vi "matlab_for_acquisition.vi"(4 "illumination last degree":dbl, 6 "illumination delay degree":dbl, 8 "dmd pattern num":dbl, 9 "camera delay degree":dbl, 10 "dmd delay degree":dbl, 11 "signal_time(ms)":dbl) -> (0 "exposure time":dbl, 1 "sample num":dbl, 2 "DO signal":dbl[][](array[numeric]), 3 "sample rate":dbl, 5 "dmd_picture_time":dbl)   [LabVIEW 2019]
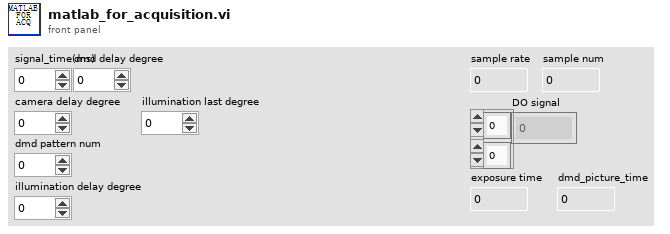
[diagram p1: front panel]
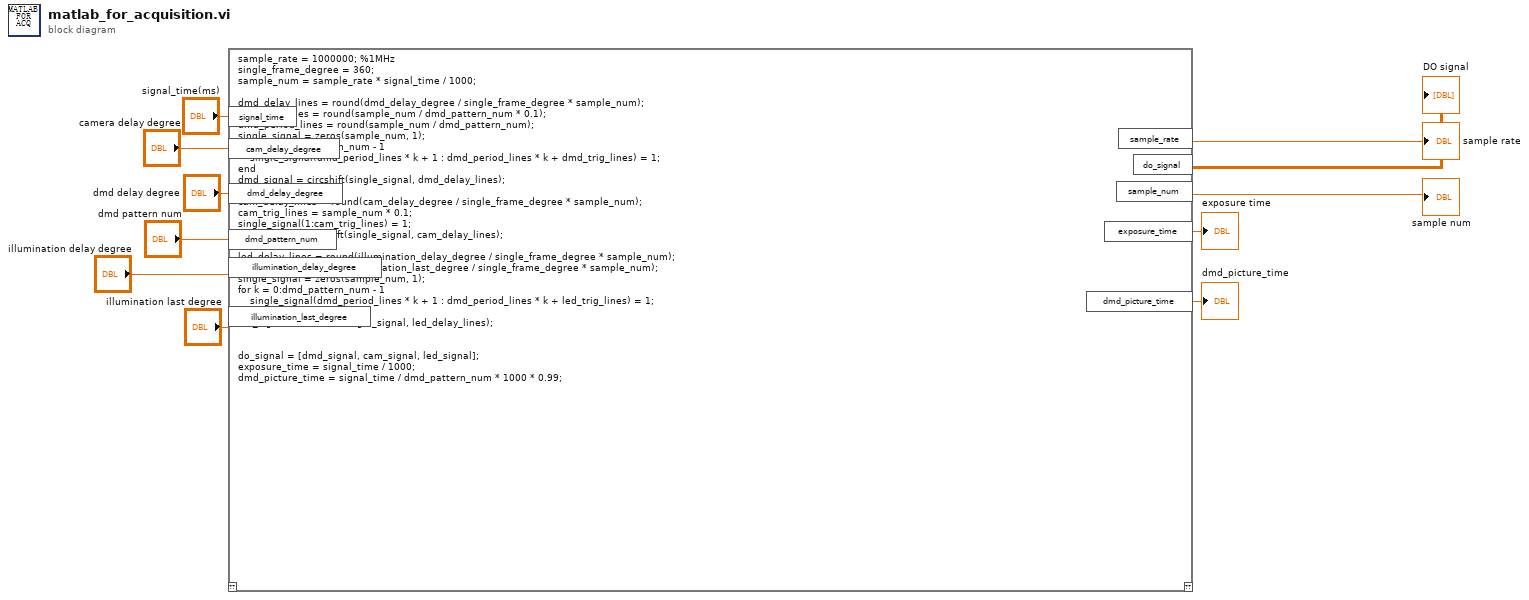
[diagram p0: block diagram]
diagram:
  n1 = script code="sample_rate = 1000000; %1MHz\nsingle_frame_degree = 360;\nsample_num = sample_rate * signal_time / 1000;\n\ndmd_delay_lines = round(dmd_delay_degree / single_frame_degree * sample_num);\ndmd_trig_lines = round(sample_num / dmd_pattern_num * 0.1);\ndmd_period_lines = round(sample_num / dmd_pattern_num);\nsingle_signal = zeros(sample_num, 1);\nfor k = 0:dmd_pattern_num - 1\n    single_signal(dmd_period_lines * k + 1 : dmd_period_lines * k + dmd_trig_lines) = 1;\nend\ndmd_signal = circshift(single_signal, dmd_delay_lines);\n\ncam_delay_lines = round(cam_delay_degree / single_frame_degree * sample_num);\ncam_trig_lines = sample_num * 0.1;\nsingle_signal(1:cam_trig_lines) = 1;\ncam_signal = circshift(single_signal, cam_delay_lines);\n\nled_delay_lines = round(illumination_delay_degree / single_frame_degree * sample_num);\nled_trig_lines = round(illumination_last_degree / single_frame_degree * sample_num);\nsingle_signal = zeros(sample_num, 1);\nfor k = 0:dmd_pattern_num - 1\n    single_signal(dmd_period_lines * k + 1 : dmd_period_lines * k + led_trig_lines) = 1;\nend\nled_signal = circshift(single_signal, led_delay_lines);\n\n\ndo_signal = [dmd_signal, cam_signal, led_signal];\nexposure_time = signal_time / 1000;\ndmd_picture_time = signal_time / dmd_pattern_num * 1000 * 0.99;"("signal_time"="signal_time(ms)", "cam_delay_degree"="camera delay degree", "dmd_delay_degree"="dmd delay degree", "dmd_pattern_num"="dmd pattern num", "illumination_delay_degree"="illumination delay degree", "illumination_last_degree"="illumination last degree") -> ("do_signal"=→"DO signal":dbl[][], "sample_rate"=→"sample rate":dbl, "sample_num"=→"sample num":dbl, "exposure_time"=→"exposure time":dbl, "dmd_picture_time"=→"dmd_picture_time":dbl)  [unwired: 1 in, 1 out]
